vi "Pre Launch Init.vi"(11 "User Interface in":refnum<class "User Interface.lvclass">) -> (0 "error out":errorcluster, 3 "User Interface out":refnum<class "User Interface.lvclass">)   [LabVIEW 2022 SP3, in "User Interface.lvlib" / "User Interface.lvclass"]
doc: "(<B>Filename</B>: Actor Framework.lvlib:Actor.lvclass:Pre Launch Init.vi)\n\nDefines behavior that occurs after the Launch Actor method is invoked but before the actor's Actor Core method begins running.\n\nThe Pre Launch Init method is guaranteed to finish before the Launch Actor method returns to its caller and before the actor itself receives any messages. Any references that the Pre Launch Init method obtains are guaranteed to have the same lifetime as the actor itself. Any errors that the Pre Launch Init method returns will abort the launch.\n\nBy default, this method does nothing. A descendant class may override it to define behavior."
uses:
  User Interface.lvclass
  User Interface.lvclass/User Interface.ctl
  <vilib>/ActorFramework/Actor/Actor.lvclass
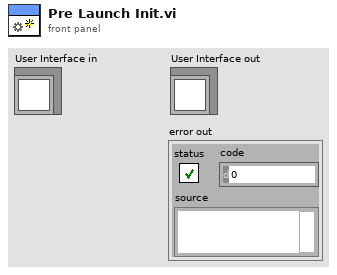
[diagram p1: front panel]
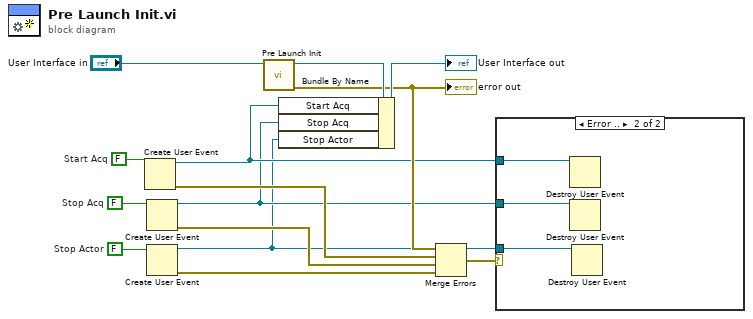
[diagram p0: block diagram]
diagram:
  w3 = FALSE  # Stop Actor
  w11 = FALSE  # Stop Acq
  w12 = FALSE  # Start Acq
  n1 = Create User Event(user event datatype=w12) -> (user event=w5:refnum<user-event>, error out=w8:errorcluster)  [unwired: 1 in]
  n2 = Create User Event(user event datatype=w11) -> (user event=w4:refnum<user-event>, error out=w9:errorcluster)  [unwired: 1 in]
  n3 = Create User Event(user event datatype=w3) -> (user event=w2:refnum<user-event>, error out=w1:errorcluster)  [unwired: 1 in]
  n4 = call-parent "Pre Launch Init.vi"("Actor in"="User Interface in") -> ("error out"=w7:errorcluster, "Actor out"=w14:refnum<class "User Interface.lvclass">)  [unwired: 9 in]
  "error out" <- w7
  n5 = Bundle By Name(cluster=w14, "Start Acq"=w5, "Stop Acq"=w4, "Stop Actor"=w2) -> (→"User Interface out":refnum<class "User Interface.lvclass">)
  n6 = Merge Errors(w7, w8, w9, w1) -> (w6:errorcluster)
  n7 = case shown="Error .." w6 {
    tunnel: w5 -> [_ w17]
    tunnel: w4 -> [_ w16]
    tunnel: w2 -> [_ w15]
    frame No Error {
    }
    frame Error {
      n8 = Destroy User Event(user event=w17) -> ()  [unwired: 1 in, 1 out]
      n9 = Destroy User Event(user event=w16) -> ()  [unwired: 1 in, 1 out]
      n10 = Destroy User Event(user event=w15) -> ()  [unwired: 1 in, 1 out]
    }
  }
